vi "ResolveSymbolicPath.vi"(11 "path":path) -> (3 "File Path":path)   [LabVIEW 2020, in "DependencyChecker.lvlib"]
uses:
  DependencyChecker.lvlib
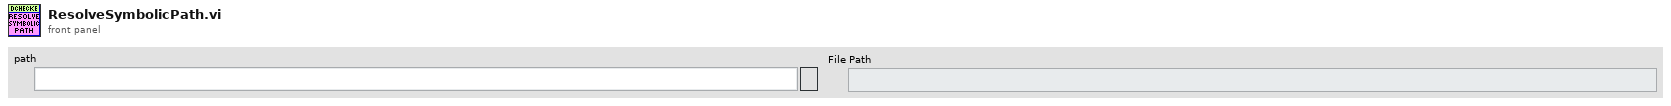
[diagram p1: front panel]
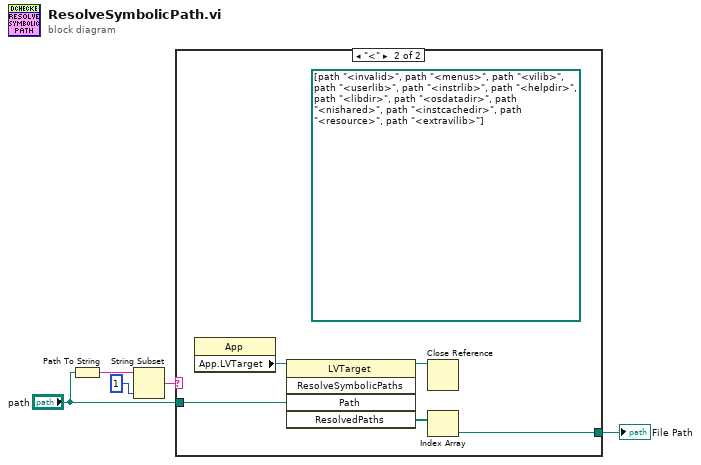
[diagram p0: block diagram]
diagram:
  n1 = Path To String(path="path") -> (string=w5:string)
  n2 = String Subset(string=w5, length (rest)=1 ("length (rest)")) -> (substring=w3:string)  [unwired: 1 in]
  n3 = case shown="\"<\"" w3 {
    tunnel: "path" -> [w6 w9]
    tunnel: [w6 w7] -> w1
    frame "False", Default {
    }
    frame "<" {
      (unwired) path[] [path "<invalid>", path "<menus>", path "<vilib>", path "<userlib>", path "<instrlib>", path "<helpdir>", path "<libdir>", path "<osdatadir>", path "<nishared>", path "<instcachedir>", path "<resource>", path "<extravilib>"]
      n4 = property class="App"() -> ("App.LVTarget"=w10:refnum<vi>)  [unwired: 2 in, 2 out]
      n5 = invoke class="LVTarget" method="ResolveSymbolicPaths"(reference=w10, "Path"=w9) -> (reference out=w11:refnum<vi>, "ResolvedPaths"=w8:path[])  [unwired: 3 in, 3 out]
      n6 = Close Reference(reference=w11) -> ()  [unwired: 1 in, 1 out]
      n7 = Index Array(array=w8) -> (element=w7:path)  [unwired: 1 in]
    }
  }
  "File Path" <- w1
